vi "Decode_waveform_file.vi"(4 "error in":errorcluster, 7 "Waveform file":path) -> (0 "error out":errorcluster, 1 "Marker 1 Data 2":u8[](array[numeric]), 2 "Marker 1 Data":u8[](array[numeric]), 3 "Channel Data":sgl[](array[numeric]))   [LabVIEW 2010]
panel:
  out "Waveform Length":i32
  out "header length":i32
  out "Length":i32
  out "MAGIC":i32
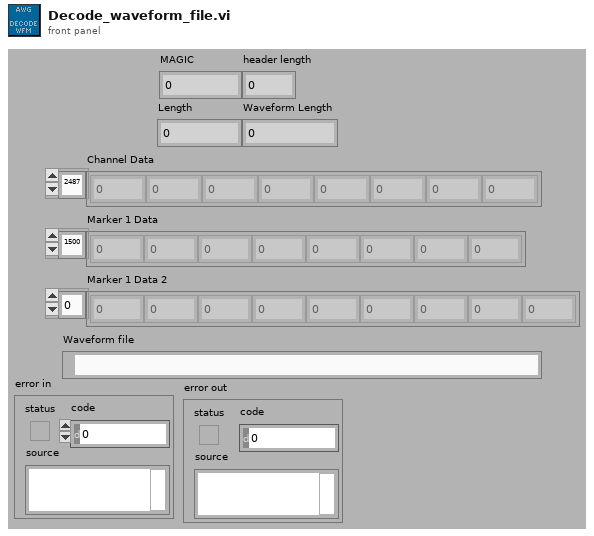
[diagram p1: front panel]
types:
  T1 = enum16{"big-endian, network order", "native, host order", "little-endian"}
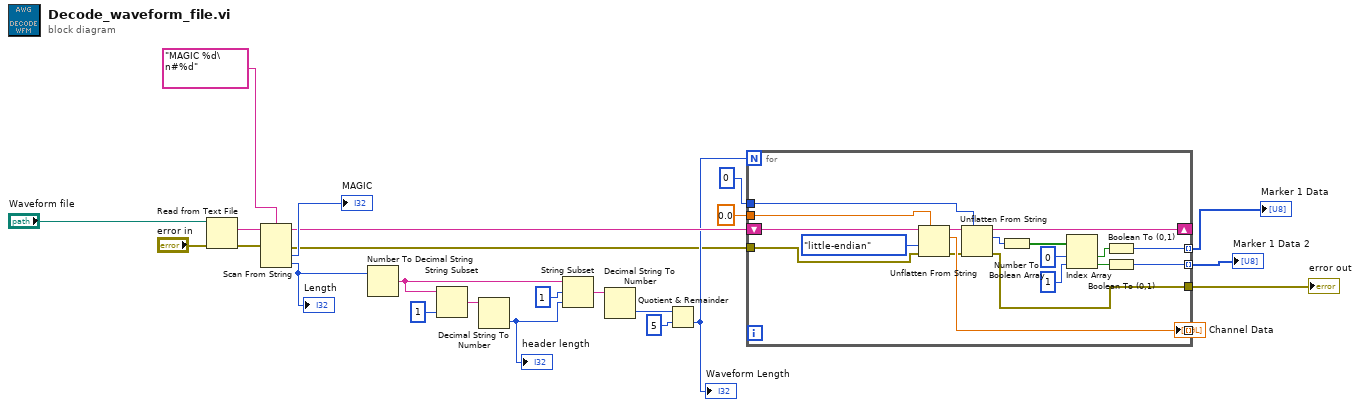
[diagram p0: block diagram]
diagram:
  n1 = Read from Text File(file (use dialog)="Waveform file", error in="error in") -> (text=w23:string, error out=w3:errorcluster)  [unwired: 2 in, 2 out]
  n2 = Scan From String(format string="MAGIC %d\n#%d", input string=w23, error in=w3) -> (remaining string=w20:string, error out=w2:errorcluster, output 1=→"MAGIC":i32, output 2=w14:i32)  [unwired: 3 in, 1 out]
  "Length" <- w14
  n3 = Number To Decimal String(number=w14) -> (decimal integer string=w11:string)  [unwired: 1 in]
  n4 = String Subset(string=w11, length (rest)=1 ("length (rest)")) -> (substring=w12:string)  [unwired: 1 in]
  n5 = Decimal String To Number(string=w12) -> (number=w9:i32)  [unwired: 2 in, 1 out]
  "header length" <- w9
  n6 = String Subset(string=w11, offset (0)=1 ("length (rest)"), length (rest)=w9) -> (substring=w8:string)
  n7 = Decimal String To Number(string=w8) -> (number=w7:i32)  [unwired: 2 in, 1 out]
  n8 = Quotient & Remainder(x=w7, y=5) -> (floor(x/y)=w5:i32)  [unwired: 1 out]
  "Waveform Length" <- w5
  n9 = for {
    N: w5 -> [_]
    shift-right: [w36] -> _
    shift-left: w20 -> [w41]
    tunnel: sgl 0.0 -> [w40]
    tunnel: [w39] -> w18 mode=indexing
    tunnel: u8 0 -> [w37]
    tunnel: [w30] -> w16 mode=indexing
    tunnel: [w28] -> w15 mode=indexing
    tunnel: w2 -> [w25]
    tunnel: [w26] -> w1
    n10 = Unflatten From String(type=w40, binary string=w41, byte order (0:big-endian, network order)=T1."little-endian", error in (no error)=w25) -> (rest of the binary string=w38:string, value=w39:sgl, error out=w27:errorcluster)  [unwired: 1 in]
    n11 = Unflatten From String(type=w37, binary string=w38, error in (no error)=w27) -> (rest of the binary string=w36:string, value=w35:u8, error out=w26:errorcluster)  [unwired: 2 in]
    n12 = Number To Boolean Array(number=w35) -> (Boolean array=w34:bool[])
    n13 = Index Array(array=w34, index #1=0 ("index"), index #2=1 ("index")) -> (element #1=w31:bool, element #2=w29:bool)
    n14 = Boolean To (0,1)(Boolean=w31) -> (0, 1=w30:i16)
    n15 = Boolean To (0,1)(Boolean=w29) -> (0, 1=w28:i16)
  }
  "Channel Data" <- w18
  "Marker 1 Data" <- w16
  "Marker 1 Data 2" <- w15
  "error out" <- w1
